vi "Conveyer Belt Global Data.vi"() -> ()   [LabVIEW 2012]
panel:
  in  "Conv Backword":bool
  in  "Conv Forword":bool
  in  "Stack Counter":dbl
  in  "Fast Speed":dbl
  in  "Mid Speed":dbl
  in  "Slow Speed":dbl
  in  "Conveyer Belt Info":T1
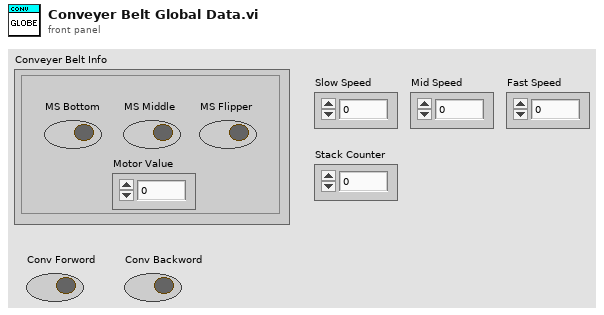
[diagram p1: front panel]
types:
  T1 = cluster{"MS Bottom":bool, "MS Middle":bool, "MS Flipper":bool, "Motor Value":dbl}
diagram:
